vi "PH_Tektronix_7000.PC Set Allow Configure.vi"(0 "i ref in":refnum<vi>, 2 "Allow Configure?":bool, 5 "error in (no error)":errorcluster) -> (14 "i ref out":refnum<vi>, 19 "error out":errorcluster)   [LabVIEW 2014, in "PH_Tektronix_7000.lvlib"]
doc: "This is the Proc Case \"Remote Control\"."
uses:
  PH_Tektronix_7000.lvlib
  PH_Common/PH_Common.lvlib
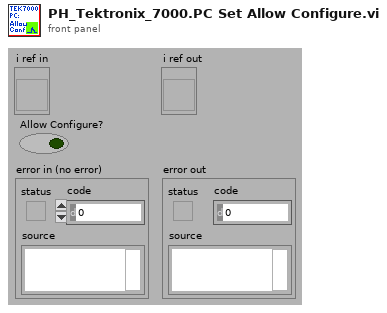
[diagram p1: front panel]
types:
  T1 = typedef "PH_Tektronix_7000.lvlib/PH_Tektronix_7000.i attribute.ctl" = cluster{"VISA Resource Name":refnum<visa-resource-name>, "IDN":cluster{"Instrument Driver":string, "Instrument Firmware":string, "Model":string, "Serial Number":string}, "Selftest":cluster{"Result":i32, "Message":string}, "Trigger Configuration":T2, "Acquisition Configuration":T3, "GUI Refs":T4, "State":T5, "Error Message":string, "Allow Prdc Loop?":bool, "Channel 1":T6, "Channel 2":T6, "Channel 3":T6, "Channel 4":T6, "Data CH 1":waveform(dbl), "Data CH 2":waveform(dbl), "Data CH 3":waveform(dbl), "Data CH 4":waveform(dbl), "Allow config?":bool, "Name Channel 1":string, "Name Channel 2":string, "Name Channel 3":string, "Name Channel 4":string, "Fetch Data before sending to PSDB?":bool, "Constructor passed?":bool, "Data taken at":timestamp, "Plot Colors":u32[], "Default VISA Resource":string}
  T2 = typedef "PH_Tektronix_7000.lvlib/PH_Tektronix_7000.Trigger Config.ctl" = cluster{"Source":u16, "Level [V]":dbl, "Slope":u16, "Coupling":u16, "Trigger Mode":u16}
  T3 = typedef "PH_Tektronix_7000.lvlib/PH_Tektronix_7000.Acquisition Config.ctl" = cluster{"Record Length":u32, "Timebase [s/div]":dbl, "Position [%]":dbl, "Acquisition Type":u16, "Average Waveforms":i32, "Envelope Waveforms":i32, "WfmDB Samples":i32, "Continuous?":bool, "Delay [s]":dbl, "Run?":bool}
  T4 = typedef "PH_Tektronix_7000.lvlib/PH_Tektronix_7000.GUI Refs.ctl" = cluster{"Graph":refnum<vi>, "State":refnum<vi>, "Delete":refnum<vi>, "VISA Resource":refnum<vi>, "Allow Configure":refnum<vi>, "Fetch Data":refnum<vi>, "Fetch before sending Data to PSDB":refnum<vi>, "Name Channel 1":refnum<vi>, "Name Channel 2":refnum<vi>, "Name Channel 3":refnum<vi>, "Name Channel 4":refnum<vi>, "Prdc Intervall [ms]":refnum<vi>, "Data taken":refnum<vi>, "Model":refnum<vi>, "Serial Number":refnum<vi>, "Firmware":refnum<vi>, "Driver":refnum<vi>, "Acquisition":refnum<vi>, "Trigger":refnum<vi>, "Cursor: D Time [s]":refnum<vi>, "Cursor: D Signal [V]":refnum<vi>, "Channel 1":refnum<vi>, "Channel 2":refnum<vi>, "Channel 3":refnum<vi>, "Channel 4":refnum<vi>}
  T5 = typedef "PH_StatusHandler.lvlib/PH_StatusHandler.Status.ctl" = i16
  T6 = typedef "PH_Tektronix_7000.lvlib/PH_Tektronix_7000.Channel Config.ctl" = cluster{"Enable Channel":bool, "Bandwidth":u16, "Input Impedance":u16, "Vertical Coupling":u16, "Probe Attenuation":dbl, "Range [V/div]":dbl, "Position [div]":dbl, "Bandwidth raw":string}
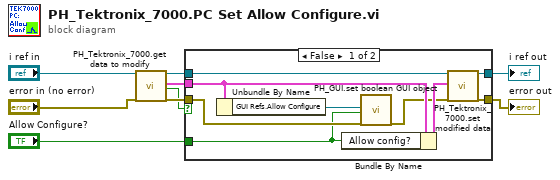
[diagram p0: block diagram]
diagram:
  n1 = call "PH_Tektronix_7000.get data to modify.vi"("i ref in"="i ref in", "error in (no error)"="error in (no error)") -> ("i ref out"=w9:refnum<vi>, "i attribute"=w5:T1, "timed out"=w3:bool, "error out"=w6:errorcluster)  [unwired: 14 in]
  n2 = case shown="False" w3 {
    tunnel: w9 -> [w18 w20]
    tunnel: [w17 w20] -> w2
    tunnel: w6 -> [w16 w19]
    tunnel: [w15 w19] -> w1
    tunnel: w5 -> [w14 _]
    tunnel: "Allow Configure?" -> [w11 _]
    frame False {
      n3 = Unbundle By Name(w14) -> ("GUI Refs.Allow Configure"=w10:refnum<vi>)
      n4 = Bundle By Name(cluster=w14, "Allow config?"=w11) -> (w13:T1)
      n5 = call "PH_GUI.set boolean GUI object.vi"("Boolean Knob GUI Ref"=w10, "Value"=w11, "error in (no error)"=w16) -> ("error out"=w12:errorcluster)  [unwired: 16 in]
      n6 = call "PH_Tektronix_7000.set modified data.vi"("i ref in"=w18, "i attribute"=w13, "error in (no error)"=w12) -> ("i ref out"=w17:refnum<vi>, "error out"=w15:errorcluster)  [unwired: 15 in]
    }
    frame True {
    }
  }
  "i ref out" <- w2
  "error out" <- w1
